vi "FPGA (Top Level - Parallax).vi"() -> ()   [LabVIEW 2017]
uses:
  <vilib>/LabVIEW Targets/FPGA/cRIO/cRIO-9505/controls.llb/_nicrio_cRIO-9505_DriveStatus.ctl
  <vilib>/Platform/TimedLoop/XDataNode/timing_clust.ctl
  <vilib>/Platform/TimedLoop/XDataNode/nitl_modes.ctl
  <vilib>/Platform/TimedLoop/XDataNode/wakeup.ctl
  <vilib>/rvi/FXPMathLib/FxpSinAndCos/subVIs/nifxpmath_SinAndCos_SimConfig.ctl
  <vilib>/rvi/Emulation/niFpgaGetClockAttributes.vi
  <vilib>/rvi/Emulation/niFpgaSctlEmulationGetInTimedLoop.vi
  <vilib>/rvi/Emulation/niFpgaEmulationReportErrorSimple.vi
  <vilib>/rvi/eio/common/nirviEmuTemplateMethod_errors.vi
  <vilib>/rvi/Emulation/niFpgaEmulationIsFPGAContextNoSignature.vi
  <vilib>/rvi/DataTransferAndStorage/Container/Common/niFpgaContainerGetUniqueNameForEmu.vi
  <vilib>/rvi/Memory/Memory_Emulation/niFpgaMemoryEmulationCacheClearOnFirstRun.vi
  <vilib>/rvi/Memory/Memory_Emulation/nirvimemoryEmulationManagerCache_MakeExclusive.vi
  <vilib>/rvi/Memory/Memory_Emulation/niFpgaMemoryEmulationValidateCache.vi
  <vilib>/rvi/Memory/Memory_Emulation/nirvimemoryEmulationManagerCache_InsertValue.vi
  <vilib>/Utility/error.llb/Clear Errors.vi
  <vilib>/rvi/Memory/Memory_Emulation/nirvimemoryEmulationManagerCache_ReleaseExclusive.vi
  <vilib>/rvi/Memory/Memory_Emulation/nirvimemoryEmulationManagerCache_GetValue.vi
  <vilib>/rvi/Memory/Memory_Emulation/nirvimemoryEmulationManagerCache_SetValue.vi
  <vilib>/rvi/Emulation/niFpgaProcessEmulError.vi
  <vilib>/rvi/Emulation/niFpgaCriticalErrorInLSC.vi
  <vilib>/rvi/FXPMathLib/FxpSinAndCos/simVIs/DllFxpSinAndCosTemp_sub.vi
  <vilib>/eio/EIONode/EIONode.xnode
  <vilib>/rvi/DataTransferAndStorage/Container/XNode/niFpgaContainer.xnode
  <vilib>/rvi/DataTransferAndStorage/Register/Emulation/niFpgaRegisterEmulation.vi
  <vilib>/rvi/FXPMathLib/FxpSinAndCos/XNode/nifxpmath_SinAndCos.xnode
  <vilib>/Platform/TimedLoop/XDataNode/XDataNode.xnode
  <vilib>/Platform/TimedLoop/XDataNode/XDNodeRunTimeDep.lvlib
  <vilib>/eio/EIOMethodNode/EIOMethodNode.xnode
panel:
  out "ENC_LOOP_PERIOD_uSec":u32
  out "LINK2_ENC_CNTS":i32
  out "LINK1_ENC_CNTS":i32
  in  "Pulse 2 Period (ticks)":i32
  in  "Pulse 1 Wait (ms)":u16=10
  out "PWM Period (ticks)":u32
  in  "Pulse 1 Period (ticks)":i32
  out "PWM Loops":i32
  out "Main Loops":i32
  out "LINK2_DRIVE_STATUS":T1
  out "LINK1_DRIVE_STATUS":T1
  in  "LINK1_LENGTH_MM":fxp<+,16,12>=2.0 format="%#_19g"
  in  "LINK2_LENGTH_MM":fxp<+,16,12>=2.0 format="%#_19g"
  in  "X_OFFSET_MM":fxp<+/-,33,15>
  in  "Y_OFFSET_MM":fxp<+/-,33,15>
  out "LINK2_Y_MM":fxp<+/-,34,16>
  out "LINK2_X_MM":fxp<+/-,34,16>
  out "LINK1_Y_MM":fxp<+/-,34,16>
  out "LINK1_X_MM":fxp<+/-,34,16>
  out "Link 1 Test Y Direction":fxp<+/-,34,16>
  out "LINK1_ENC_POS":i32
  out "LINK2_ENC_POS":i32
  out "LINK1_POT_POS":i32
  out "LINK2_POT_POS":i32
  in  "LINK1_ENC_SCALE":fxp<+,32,0>=0.09645000007003546 format="%#_32g"
  in  "LINK2_ENC_SCALE":fxp<+,32,0>=0.029296900611370802 format="%#_32g"
  in  "LINK1_PWM_MAX":i16
  in  "LINK2_PWM_MAX":i16
  in  "LINK1_DEMAND_PWM":i16
  in  "LINK2_DEMAND_PWM":i16
  in  "LINK1_POT_SCALE":fxp<+/-,32,16>
  in  "LINK1_OFFSET":fxp<+/-,16,16>
  in  "LINK2_POT_SCALE":fxp<+/-,32,16>
  in  "LINK2_OFFSET":fxp<+/-,16,16>
  in  "AI_POT_LOOP_US":u16=10
  in  "ENC_DEBOUNCE_CYCLES":u16=5
  in  "LINK1_ENC_CNTS":i32
  in  "LINK2_ENC_CNTS":i32
  in  "LINK1_UPDATE_ENC":bool
  in  "LINK2_UPDATE_ENC":bool
  # "PWM at 50kHz"
  # "3.3V"
  # "10MHz Loops Rate"
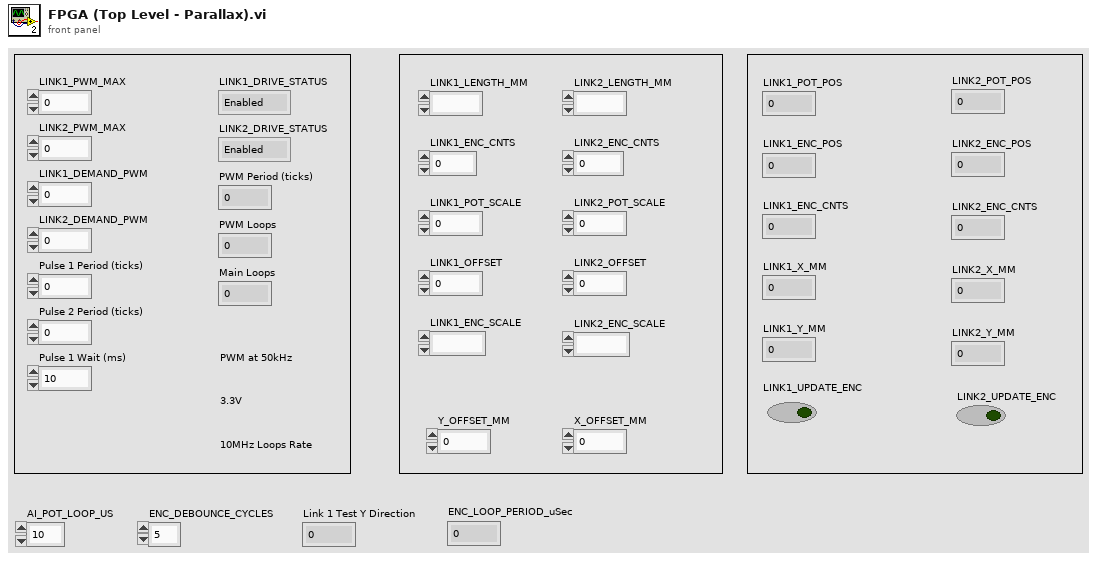
[diagram p1: front panel]
types:
  T1 = typedef "_nicrio_cRIO-9505_DriveStatus.ctl" = enum8{"Enabled", "Disabled", "Disabled by Drive Fault", "Disabled by Temp. Fault", "Disabled by E-Stop", "Unknown"}
  T2 = typedef "XDNodeRunTimeDep.lvlib/timing_clust.ctl" = cluster{"Expected End [f-1]":u64, "Actual End [f-1]":u64, "Finished Late? [f-1]":bool, "Expected End [i-1]":u64, "Actual End [i-1]":u64, "Finished Late? [i-1]":bool, "Expected Start [i]":u64, "Actual Start [i]":u64, "Expected Start [f]":u64, "Actual Start [f]":u64, "Source Name":string, "Structure Name":string, "Period":i64, "Deadline":i64, "Offset":i64, "Start":i64, "Priority":i32, "Timeout":i32, "Mode":T3, "Wakeup Reason":T4, "Error":errorcluster, "Source Type":string, "Secondary Source Type":string, "Global End Time":u64, "Global Start Time":u64, "Frame Duration":u64, "Iteration Duration":u64, "Assigned CPU":i32, "I/O Scan Engine Mode":u32}
  T3 = typedef "XDNodeRunTimeDep.lvlib/nitl_modes.ctl" = enum32{"No Change", "Process missed periods, maintain original phase", "Discard missed periods, maintain original phase", "Process missed periods, ignore original phase", "Discard missed periods, ignore original phase"}
  T4 = typedef "XDNodeRunTimeDep.lvlib/wakeup.ctl" = enum32{"Normal", "Aborted", "Asynchronous wakeup", "Timing source error", "Timed loop error", "Timeout"}
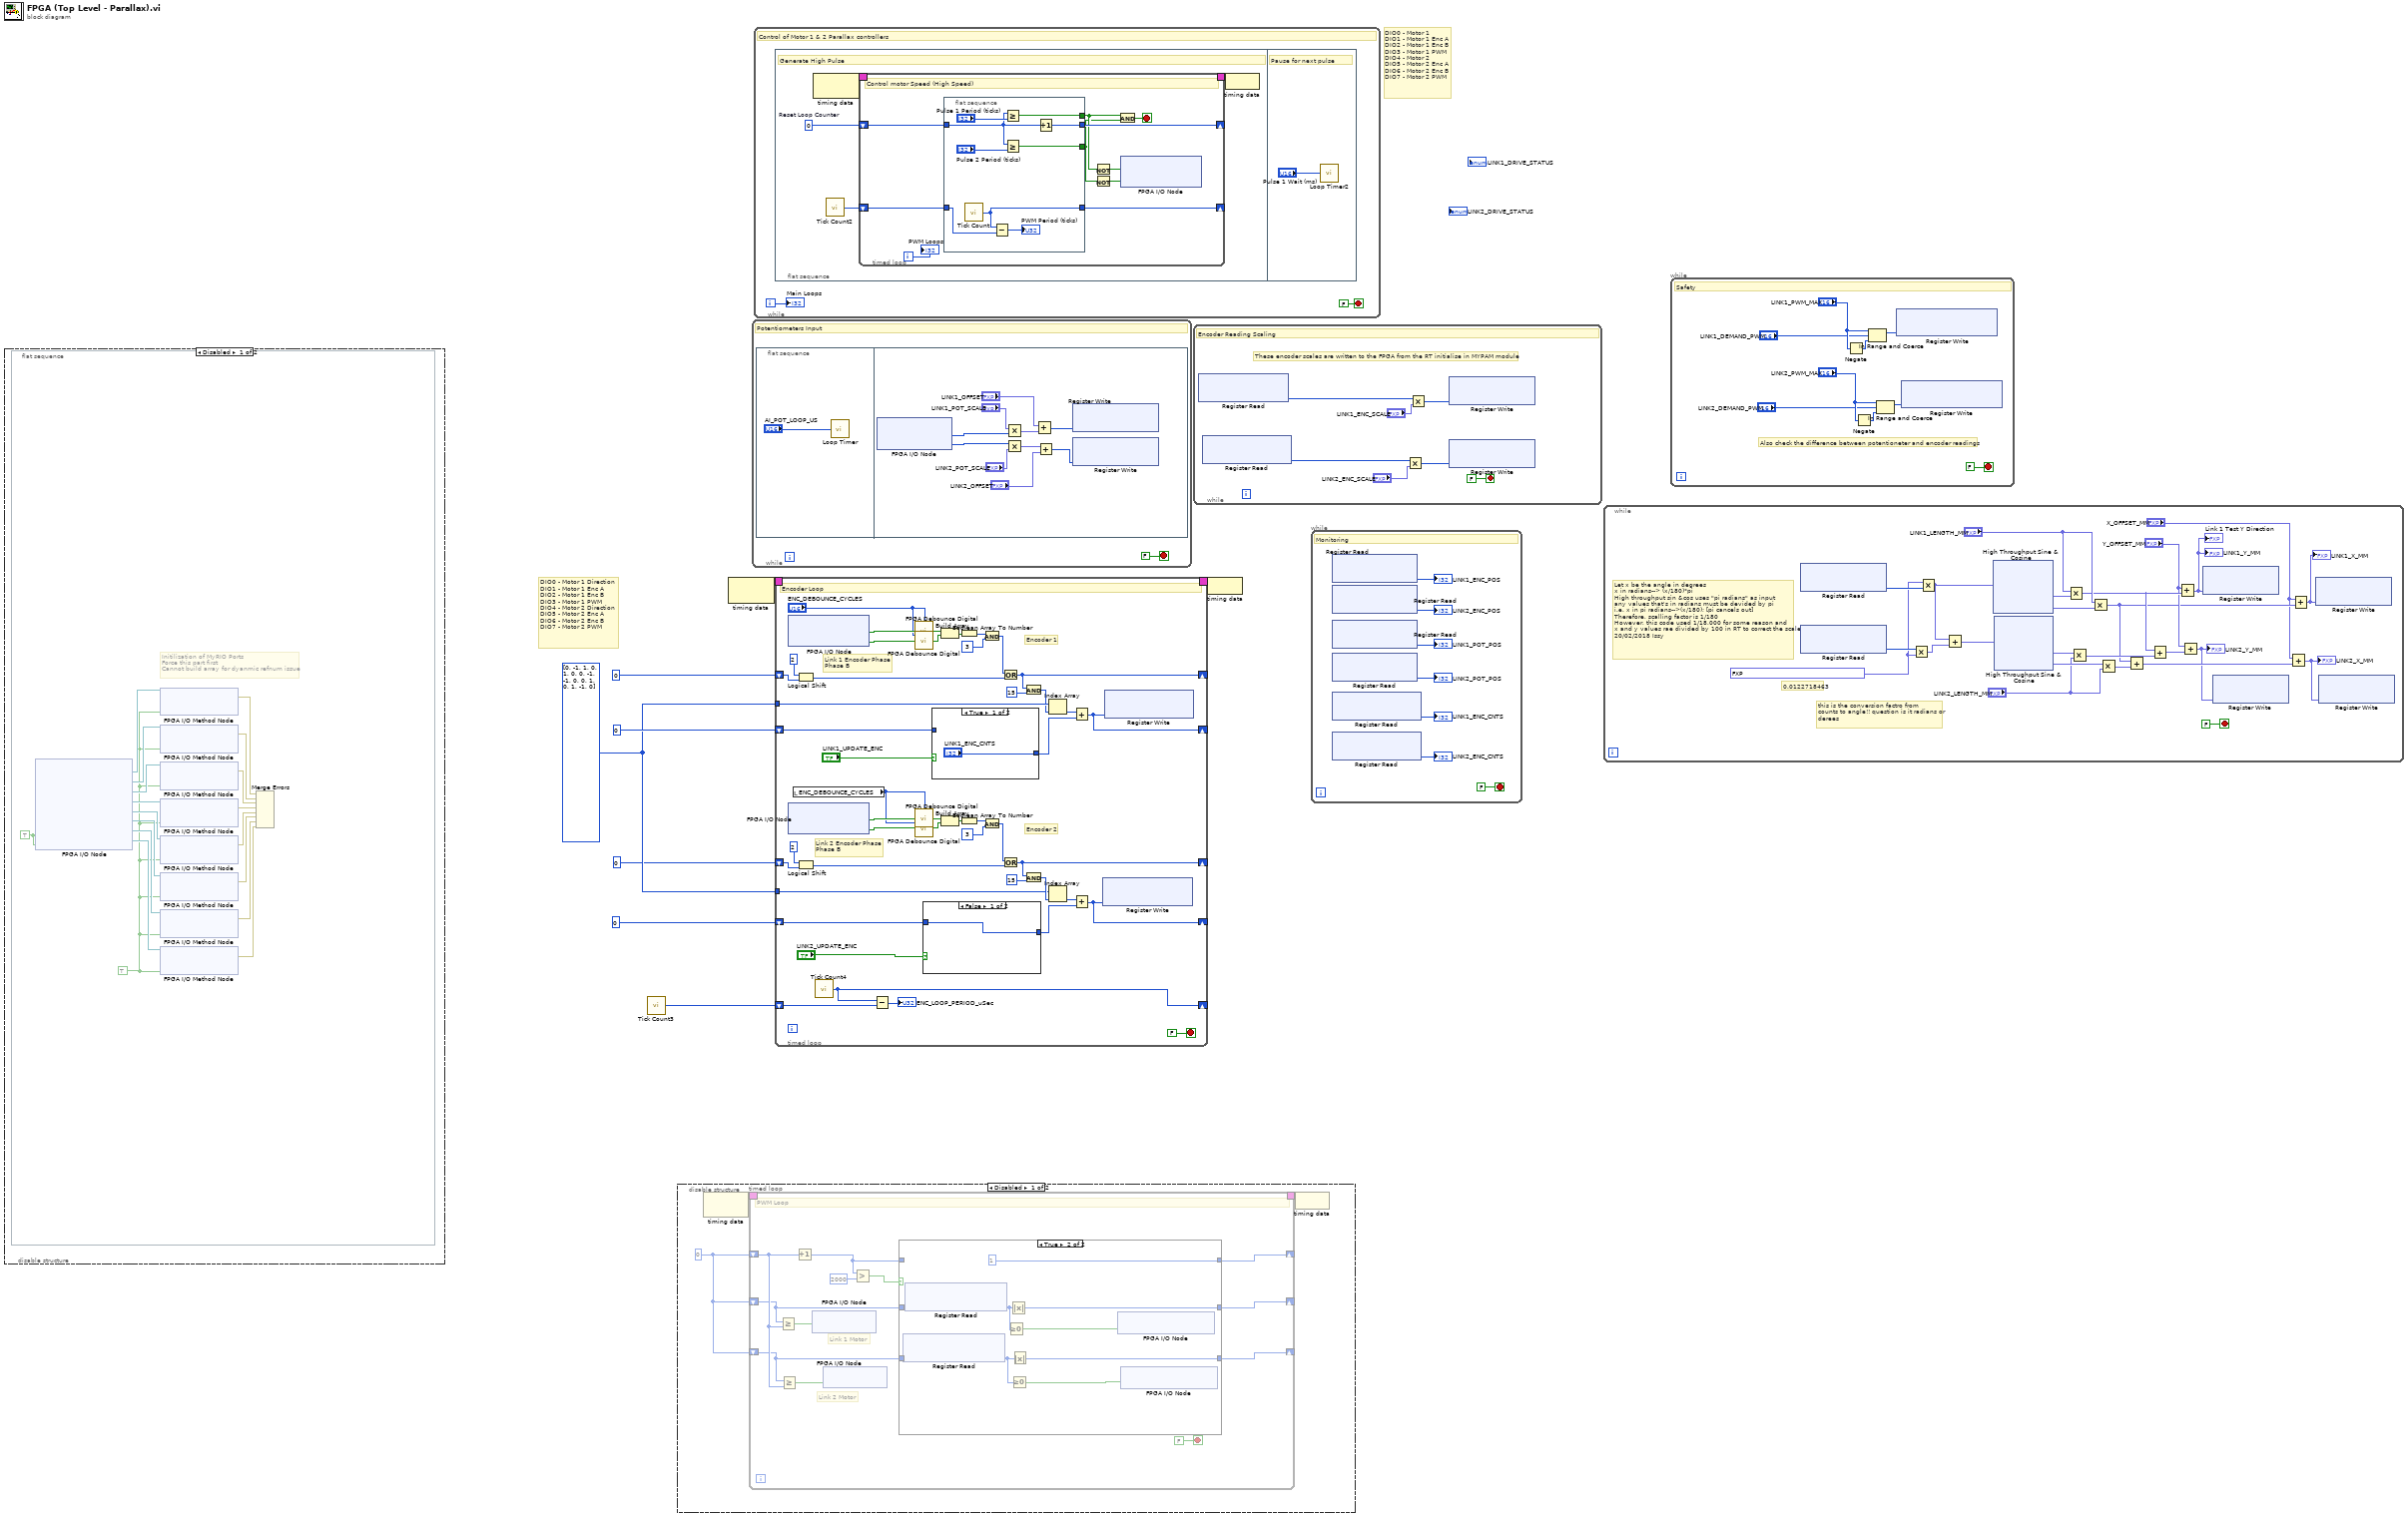
[diagram p0: block diagram]
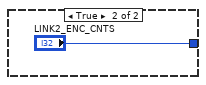
[diagram p5: hidden frame]
diagram:
  w4 = i8[] [0, -1, 1, 0, 1, 0, 0, -1, -1, 0, 0, 1, 0, 1, -1, 0]
  # "DIO0 - Motor 1 Direction \nDIO1 - Motor 1 Enc A\nDIO2 - Motor 1 Enc B\nDIO3 - Motor 1 PWM\nDIO4 - Motor 2 Direction\nDIO5 - Motor 2 Enc A\nDIO6 - Motor 2 Enc B\nDIO7 - Motor 2 PWM"
  # "DIO0 - Motor 1  \nDIO1 - Motor 1 Enc A\nDIO2 - Motor 1 Enc B\nDIO3 - Motor 1 PWM\nDIO4 - Motor 2 \nDIO5 - Motor 2 Enc A\nDIO6 - Motor 2 Enc B\nDIO7 - Motor 2 PWM"
  n1 = disable-structure shown="Disabled" {
    frame Disabled {
      n2 = flat-sequence {
        frame #0 {
          w17 = TRUE ("Link 2 Encoder Phase B")
          w26 = TRUE ("Link 2 Encoder Phase B")
          # "Initilization of MyRIO Ports\nForce this part first \nCannot build array for dyanmic refnum issue"
          n3 = xnode "FPGA I/O Node"("Link 2 Encoder Phase B"=w26, "Motor 2 Drive Direction"=w26) -> ("FPGA I/O Out"=w25:refnum<k21>, "FPGA I/O Out"=w24:refnum<k21>, "FPGA I/O Out"=w23:refnum<k21>, "FPGA I/O Out"=w22:refnum<k21>, "FPGA I/O Out"=w21:refnum<k21>, "FPGA I/O Out"=w20:refnum<k21>, "FPGA I/O Out"=w19:refnum<k21>, "FPGA I/O Out"=w18:refnum<k21>)  [unwired: 8 in, 6 out]
          n4 = xnode "FPGA I/O Method Node"("FPGA I/O In"=w25, "Enable"=w17) -> ("error out"=w16:errorcluster)  [unwired: 1 in, 1 out]
          n5 = xnode "FPGA I/O Method Node"("FPGA I/O In"=w24, "Enable"=w17) -> ("error out"=w15:errorcluster)  [unwired: 1 in, 1 out]
          n6 = xnode "FPGA I/O Method Node"("FPGA I/O In"=w23, "Enable"=w17) -> ("error out"=w14:errorcluster)  [unwired: 1 in, 1 out]
          n7 = xnode "FPGA I/O Method Node"("FPGA I/O In"=w22, "Enable"=w17) -> ("error out"=w13:errorcluster)  [unwired: 1 in, 1 out]
          n8 = xnode "FPGA I/O Method Node"("FPGA I/O In"=w21, "Enable"=w17) -> ("error out"=w12:errorcluster)  [unwired: 1 in, 1 out]
          n9 = xnode "FPGA I/O Method Node"("FPGA I/O In"=w20, "Enable"=w17) -> ("error out"=w11:errorcluster)  [unwired: 1 in, 1 out]
          n10 = xnode "FPGA I/O Method Node"("FPGA I/O In"=w19, "Enable"=w17) -> ("error out"=w10:errorcluster)  [unwired: 1 in, 1 out]
          n11 = xnode "FPGA I/O Method Node"("FPGA I/O In"=w18, "Enable"=w17) -> ("error out"=w9:errorcluster)  [unwired: 1 in, 1 out]
          n12 = Merge Errors(w16, w15, w14, w13, w12, w11, w10, w9) -> ()  [unwired: 1 out]
        }
      }
    }
    frame Enabled {
    }
  }
  n13 = call "Tick Count3"() -> ("Tick Count(uSec)"=w1:u32)
  n14 = disable-structure shown="Disabled" {
    frame Disabled {
      w27 = i16 0 ("Motor 1 PWM Duty Cycle")
      n15 = node-c288() -> (w29:T2)  [unwired: 1 in]
      n16 = timed-loop {
        timing: w29 -> [_]
        timing-out: [_] -> w28
        shift-right: [w40] -> _
        shift-left: w27 -> [w39]
        shift-right: [w38] -> _
        shift-left: w27 -> [w36]
        shift-right: [w37] -> _
        shift-left: w27 -> [w35]
        stop <- FALSE stop-if-true
        # "Link 2 Motor"
        # "Link 1 Motor"
        # "PWM Loop"
        n17 = Greater Or Equal?(x=w36, y=w39) -> (x >= y?=w31:bool)
        n18 = Greater Or Equal?(x=w35, y=w39) -> (x >= y?=w30:bool)
        n19 = Increment(x=w39) -> (x+1=w33:i16)
        n20 = xnode "FPGA I/O Node"("Link 1 Motor"=w31) -> ()  [unwired: 1 in, 1 out]
        n21 = xnode "FPGA I/O Node"("Link 2 Motor"=w30) -> ()  [unwired: 1 in, 1 out]
        n22 = Greater?(x=w33, y=i16 2000) -> (0:w34:bool)
        n23 = case shown="True" w34 {
          tunnel: w33 -> [w44 _]
          tunnel: [w44 i16 1 ("Motor 1 PWM Duty Cycle")] -> w40
          tunnel: [w43 w50] -> w38
          tunnel: [w42 w49] -> w37
          tunnel: w36 -> [w43 _]
          tunnel: w35 -> [w42 _]
          frame False {
          }
          frame True {
            n24 = xnode ("Register Read")() -> ("Data"=w47:i16)  [unwired: 1 in, 1 out]
            n25 = xnode ("Register Read")() -> ("Data"=w48:i16)  [unwired: 1 in, 1 out]
            n26 = Greater Or Equal To 0?(x=w48) -> (x >= 0?=w45:bool)
            n27 = Absolute Value(x=w48) -> (abs(x)=w50:i16)
            n28 = Greater Or Equal To 0?(x=w47) -> (x >= 0?=w46:bool)
            n29 = Absolute Value(x=w47) -> (abs(x)=w49:i16)
            n30 = xnode "FPGA I/O Node"("Motor 1 Drive Direction"=w45) -> ()  [unwired: 1 in, 1 out]
            n31 = xnode "FPGA I/O Node"("Motor 2 Drive Direction"=w46) -> ()  [unwired: 1 in, 1 out]
          }
        }
      }
      n32 = node-c288(w28) -> ()
    }
    frame Enabled {
    }
  }
  n33 = node-c288() -> (w8:T2)  [unwired: 1 in]
  n34 = while {
    stop <- FALSE stop-if-true
    # "Potentiometers Input"
    n35 = flat-sequence {
      frame #0 {
        n36 = call "Loop Timer"("Count(uSec)"="AI_POT_LOOP_US") -> ()  [unwired: 1 out]
      }
      frame #1 {
        n37 = xnode "FPGA I/O Node"() -> ("ConnectorC/AI0"=w59:i16, "ConnectorC/AI1"=w58:i16)  [unwired: 2 in, 2 out]
        n38 = Multiply(x="LINK1_POT_SCALE", y=w59) -> (x*y=w66:fxp<+/-,48,32>)
        n39 = Multiply(x=w58, y="LINK2_POT_SCALE") -> (x*y=w62:fxp<+/-,48,32>)
        n40 = Add(x="LINK1_OFFSET", y=w66) -> (x+y=w60:i32)
        n41 = Add(x=w62, y="LINK2_OFFSET") -> (x+y=w61:i32)
        n42 = xnode ("Register Write")("Data"=w60) -> ()  [unwired: 1 in, 1 out]
        n43 = xnode ("Register Write")("Data"=w61) -> ()  [unwired: 1 in, 1 out]
      }
    }
  }
  n44 = while {
    i -> [w68]
    stop <- FALSE stop-if-true
    # "Control of Motor 1 & 2 Parallax controllers"
    n45 = flat-sequence {
      frame #0 {
        w70 = 0  # Reset Loop Counter
        # "Generate High Pulse"
        n46 = node-c288() -> (w73:T2)  [unwired: 1 in]
        n47 = call "Tick Count2"() -> ("Tick Count(Ticks)"=w71:u32)
        n48 = timed-loop {
          shift-right: [w83] -> _
          shift-left: w71 -> [w82]
          timing: w73 -> [_]
          timing-out: [_] -> w72
          shift-right: [w81] -> _
          shift-left: w70 -> [w80]
          i -> [w79]
          stop <- w76 stop-if-true
          # "Control motor Speed (High Speed)"
          n49 = flat-sequence {
            tunnel: [w92] -> w83
            tunnel: [w89] -> w81
            tunnel: w82 -> [w91]
            tunnel: w80 -> [w86]
            tunnel: [w88] -> w75
            tunnel: [w84] -> w74
            frame #0 {
              n50 = call "Tick Count"() -> ("Tick Count(Ticks)"=w92:u32)
              n51 = Subtract(x=w92, y=w91) -> (x-y=→"PWM Period (ticks)":u32)
              n52 = Greater Or Equal?(x=w86, y="Pulse 1 Period (ticks)") -> (x >= y?=w88:bool)
              n53 = Greater Or Equal?(x=w86, y="Pulse 2 Period (ticks)") -> (x >= y?=w84:bool)
              n54 = Increment(x=w86) -> (x+1=w89:i32)
            }
          }
          n55 = Not(x=w75) -> (.not. x?=w77:bool)
          n56 = Not(x=w74) -> (.not. x?=w78:bool)
          n57 = And(x=w75, y=w74) -> (x .and. y?=w76:bool)
          n58 = xnode "FPGA I/O Node"("ConnectorC/DIO3"=w77, "ConnectorC/DIO7"=w78) -> ()  [unwired: 2 in, 2 out]
          "PWM Loops" <- w79
        }
        n59 = node-c288(w72) -> ()
      }
      frame #1 {
        # "Pause for next pulse"
        n60 = call "Loop Timer2"("Count(mSec)"="Pulse 1 Wait (ms)") -> ()  [unwired: 1 out]
      }
    }
    "Main Loops" <- w68
  }
  n61 = timed-loop {
    timing: w8 -> [_]
    timing-out: [_] -> w7
    tunnel: w4 -> [w140]
    shift-right: [w133] -> _
    shift-left: u8 0 -> [w142]
    shift-right: [w104] -> _
    shift-left: 0 -> [w125]
    tunnel: w4 -> [w109]
    shift-right: [w107] -> _
    shift-left: u8 0 -> [w108]
    shift-right: [w103] -> _
    shift-left: 0 -> [w101]
    shift-right: [w99] -> _
    shift-left: w1 -> [w100]
    stop <- FALSE stop-if-true
    # "Link 2 Encoder Phase \nPhase B"
    # "Link 1 Encoder Phase \nPhase B"
    # "Encoder 2"
    # "Encoder 1"
    # "Encoder Loop"
    n62 = xnode "FPGA I/O Node"() -> ("ConnectorC/DIO1"=w131:bool, "ConnectorC/DIO2"=w130:bool)  [unwired: 2 in, 2 out]
    n63 = xnode "FPGA I/O Node"() -> ("ConnectorC/DIO5"=w115:bool, "ConnectorC/DIO6"=w114:bool)  [unwired: 2 in, 2 out]
    n64 = local read "ENC_DEBOUNCE_CYCLES"() -> (w106:u16)
    n65 = Logical Shift(y=i16 2, x=w142) -> (x << y=w135:u8)
    n66 = Logical Shift(y=i16 2, x=w108) -> (x << y=w118:u8)
    n67 = call "Tick Count4"() -> ("Tick Count(uSec)"=w99:u32)
    n68 = Subtract(x=w99, y=w100) -> (x-y=→"ENC_LOOP_PERIOD_uSec":u32)
    n69 = call "FPGA Debounce Digital.vi"("Input Signal"=w131, "Cycles to Filter"="ENC_DEBOUNCE_CYCLES") -> ("Output Filtered Signal"=w129:bool)
    n70 = call "FPGA Debounce Digital.vi"("Input Signal"=w130, "Cycles to Filter"="ENC_DEBOUNCE_CYCLES") -> ("Output Filtered Signal"=w128:bool)
    n71 = call "FPGA Debounce Digital.vi"("Input Signal"=w115, "Cycles to Filter"=w106) -> ("Output Filtered Signal"=w113:bool)
    n72 = call "FPGA Debounce Digital.vi"("Input Signal"=w114, "Cycles to Filter"=w106) -> ("Output Filtered Signal"=w112:bool)
    n73 = case shown="False" "LINK2_UPDATE_ENC" {
      tunnel: w101 -> [w144 _]
      tunnel: [w144 "LINK2_ENC_CNTS"] -> w110
      frame False {
      }
      frame True {
      }
    }
    n74 = case shown="True" "LINK1_UPDATE_ENC" {
      tunnel: w125 -> [_ w147]
      tunnel: ["LINK1_ENC_CNTS" w147] -> w124
      frame True {
      }
      frame False {
      }
    }
    n75 = Build Array(w129, w128) -> (w127:bool[])
    n76 = Build Array(w113, w112) -> (w111:bool[])
    n77 = Boolean Array To Number(Boolean array=w127) -> (number=w138:u8)
    n78 = Boolean Array To Number(Boolean array=w111) -> (number=w121:u8)
    n79 = And(x=w138, y=u8 3) -> (x .and. y?=w136:u8)
    n80 = And(x=w121, y=u8 3) -> (x .and. y?=w119:u8)
    n81 = Or(x=w136, y=w135) -> (x .or. y?=w133:u8)
    n82 = Or(x=w119, y=w118) -> (x .or. y?=w107:u8)
    n83 = And(x=w133, y=u8 15) -> (x .and. y?=w134:u8)
    n84 = And(x=w107, y=u8 15) -> (x .and. y?=w117:u8)
    n85 = Index Array(array=w140, index=w134) -> (element=w132:i8)
    n86 = Index Array(array=w109, index=w117) -> (element=w116:i8)
    n87 = Add(x=w132, y=w124) -> (x+y=w104:i32)
    n88 = Add(x=w116, y=w110) -> (x+y=w103:i32)
    n89 = xnode ("Register Write")("Data"=w103) -> ()  [unwired: 1 in, 1 out]
    n90 = xnode ("Register Write")("Data"=w104) -> ()  [unwired: 1 in, 1 out]
  }
  n91 = while {
    stop <- FALSE stop-if-true
    # "These encoder scales are written to the FPGA from the RT initialise in MYPAM module"
    # "Encoder Reading Scaling"
    n92 = xnode ("Register Read")() -> ("Data"=w154:i32)  [unwired: 1 in, 1 out]
    n93 = xnode ("Register Read")() -> ("Data"=w155:i32)  [unwired: 1 in, 1 out]
    n94 = Multiply(x=w155, y="LINK2_ENC_SCALE") -> (x*y=w152:i32)
    n95 = Multiply(x=w154, y="LINK1_ENC_SCALE") -> (x*y=w153:i32)
    n96 = xnode ("Register Write")("Data"=w153) -> ()  [unwired: 1 in, 1 out]
    n97 = xnode ("Register Write")("Data"=w152) -> ()  [unwired: 1 in, 1 out]
  }
  n98 = node-c288(w7) -> ()
  n99 = while {
    stop <- FALSE stop-if-true
    # "Monitoring"
    n100 = xnode ("Register Read")() -> ("Data"=→"LINK1_ENC_POS":i32)  [unwired: 1 in, 1 out]
    n101 = xnode ("Register Read")() -> ("Data"=→"LINK2_ENC_POS":i32)  [unwired: 1 in, 1 out]
    n102 = xnode ("Register Read")() -> ("Data"=→"LINK1_POT_POS":i32)  [unwired: 1 in, 1 out]
    n103 = xnode ("Register Read")() -> ("Data"=→"LINK2_POT_POS":i16)  [unwired: 1 in, 1 out]
    n104 = xnode ("Register Read")() -> ("Data"=→"LINK1_ENC_CNTS":i32)  [unwired: 1 in, 1 out]
    n105 = xnode ("Register Read")() -> ("Data"=→"LINK2_ENC_CNTS":i32)  [unwired: 1 in, 1 out]
  }
  n106 = while {
    stop <- FALSE stop-if-true
    w164 = fxp<+,32,-7> 5.55555998289492e-05
    # "Let x be the angle in degrees\nx in radians--> (x/180)*pi\nHigh throughput sin &cos uses \"pi radians\" as input\nany values that's in radians must be devided by pi\ni.e. x in pi radians-->(x/180); [pi cancels out]\nTherefore, scalling factor is 1/180\nHowever, this code used 1/18,000 for some reason and\nx and y values rae divided by 100 in RT to correct the scale.\n20/02/2018 Issy"
    # "0.0122718463"
    # "this is the conversion factro from \ncounts to angle!! question is it radians or\nderees"
    n107 = xnode ("Register Read")() -> ("Data"=w170:i32)  [unwired: 1 in, 1 out]
    n108 = xnode ("Register Read")() -> ("Data"=w187:i32)  [unwired: 1 in, 1 out]
    n109 = Multiply(x=w187, y=w164) -> (x*y=w186:fxp<+/-,64,25>)
    n110 = Multiply(x=w164, y=w170) -> (x*y=w169:fxp<+/-,64,25>)
    n111 = Add(x=w169, y=w186) -> (x+y=w185:fxp<+/-,64,26>)
    n112 = xnode "High Throughput Sine & Cosine"("x (pi)"=w169) -> ("sin(x)"=w184:fxp<+/-,16,2>, "cos(x)"=w183:fxp<+/-,16,2>)
    n113 = xnode "High Throughput Sine & Cosine"("x (pi)"=w185) -> ("sin(x)"=w181:fxp<+/-,16,2>, "cos(x)"=w180:fxp<+/-,16,2>)
    n114 = Multiply(x="LINK1_LENGTH_MM", y=w184) -> (x*y=w176:fxp<+/-,32,14>)
    n115 = Multiply(x=w181, y="LINK2_LENGTH_MM") -> (x*y=w177:fxp<+/-,32,14>)
    n116 = Multiply(x="LINK1_LENGTH_MM", y=w183) -> (x*y=w173:fxp<+/-,32,14>)
    n117 = Multiply(x=w180, y="LINK2_LENGTH_MM") -> (x*y=w178:fxp<+/-,32,14>)
    n118 = Add(x=w173, y=w178) -> (x+y=w172:fxp<+/-,33,15>)
    n119 = Add(x=w176, y=w177) -> (x+y=w175:fxp<+/-,33,15>)
    n120 = Add(x="Y_OFFSET_MM", y=w176) -> (x+y=w166:fxp<+/-,34,16>)
    "LINK1_Y_MM" <- w166
    "Link 1 Test Y Direction" <- w166
    n121 = Add(x="Y_OFFSET_MM", y=w175) -> (x+y=w168:fxp<+/-,34,16>)
    "LINK2_Y_MM" <- w168
    n122 = xnode ("Register Write")("Data"=w166) -> ()  [unwired: 1 in, 1 out]
    n123 = xnode ("Register Write")("Data"=w168) -> ()  [unwired: 1 in, 1 out]
    n124 = Add(x="X_OFFSET_MM", y=w172) -> (x+y=w167:fxp<+/-,34,16>)
    "LINK2_X_MM" <- w167
    n125 = Add(x="X_OFFSET_MM", y=w173) -> (x+y=w165:fxp<+/-,34,16>)
    "LINK1_X_MM" <- w165
    n126 = xnode ("Register Write")("Data"=w165) -> ()  [unwired: 1 in, 1 out]
    n127 = xnode ("Register Write")("Data"=w167) -> ()  [unwired: 1 in, 1 out]
  }
  n128 = while {
    stop <- FALSE stop-if-true
    # "Also check the difference between potentioneter and encoder readings"
    # "Safety"
    n129 = Negate(x="LINK1_PWM_MAX") -> (-x=w255:i16)
    n130 = Negate(x="LINK2_PWM_MAX") -> (-x=w253:i16)
    n131 = In Range and Coerce(upper limit="LINK1_PWM_MAX", x="LINK1_DEMAND_PWM", lower limit=w255) -> (coerced(x)=w256:i16)  [unwired: 1 out]
    n132 = In Range and Coerce(upper limit="LINK2_PWM_MAX", x="LINK2_DEMAND_PWM", lower limit=w253) -> (coerced(x)=w252:i16)  [unwired: 1 out]
    n133 = xnode ("Register Write")("Data"=w256) -> ()  [unwired: 1 in, 1 out]
    n134 = xnode ("Register Write")("Data"=w252) -> ()  [unwired: 1 in, 1 out]
  }
